vi "Stop Core.vi"(10 "final error code":i32, 11 "CS++DSMonitor in":refnum<class "CS++DSMonitor.lvclass">) -> (3 "CS++DSMonitor out":refnum<class "CS++DSMonitor.lvclass">)   [LabVIEW 2016, in "CS++DSMonitor.lvlib" / "CS++DSMonitor.lvclass"]
doc: "(<B>Filename</B>: Actor Framework.lvlib:Actor.lvclass:Stop Core.vi)\n\nDefines what the actor does before it stops. Use the <B>final error code</B> input to determine whether the actor shut down in response to an error.\n\nBy default, this method does nothing. A descendant class may override it to define behavior, such as shutting down any processes the actor initiated in its override of the Actor Core method."
uses:
  CS++DSMonitor.lvclass
  CS++DSMonitor.lvclass/CS++DSMonitor.ctl
  CS++PVMonitor/CS++PVMonitor.lvclass
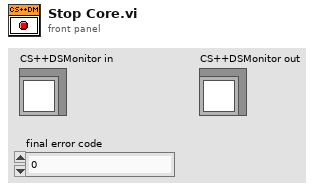
[diagram p1: front panel]
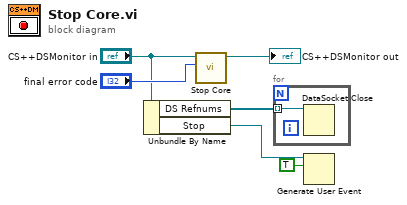
[diagram p0: block diagram]
diagram:
  n1 = Unbundle By Name("CS++DSMonitor in") -> ("DS Refnums"=w3:refnum<k13>[], "Stop"=w2:refnum<user-event>)
  n2 = call-parent "Stop Core.vi"("final error code"="final error code", "CS++BaseActor in"="CS++DSMonitor in") -> ("CS++BaseActor out"=→"CS++DSMonitor out":refnum<class "CS++DSMonitor.lvclass">)  [unwired: 9 in]
  n3 = for {
    tunnel: w3 -> [w7] mode=indexing
    n4 = DataSocket Close(11:w7) -> ()  [unwired: 2 in, 2 out]
  }
  n5 = Generate User Event(user event=w2, event data cluster=TRUE ("event data")) -> ()  [unwired: 2 in, 2 out]
